vi "Untitled 2.vi"() -> ()   [LabVIEW 2016]
uses:
  <vilib>/AppBuilder/AB_API/PPL/NI_AB_API_PPL.lvclass
  <vilib>/AppBuilder/AB_API/Build/NI_AB_API_Build.lvclass
  <vilib>/AppBuilder/AB_API/SDIST/NI_AB_API_SDIST.lvclass
  C:/Program Files (x86)/National Instruments/LabVIEW 2016/vi.lib/AppBuilder/AB_API/Targetfile/NI_AB_API_Targetfile.lvclass
  C:/Program Files (x86)/National Instruments/LabVIEW 2016/vi.lib/AppBuilder/AB_API/Build/NI_AB_API_Build.lvclass
panel:
  in  "Destination":string
  out "Primary destination path":path
  out "error out":errorcluster
  out "Cluster":cluster{string, "Build":string, string}
  in  "Cancel":bool
  in  "OK":bool
  in  "Build":string(combo)
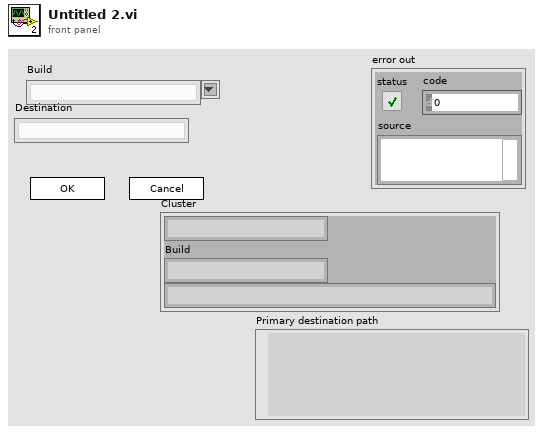
[diagram p1: front panel]
types:
  T1 = enum8{"Enabled", "Disabled", "Disabled and Grayed Out"}
  T2 = cluster{string, "Build":string, "Destination":string}
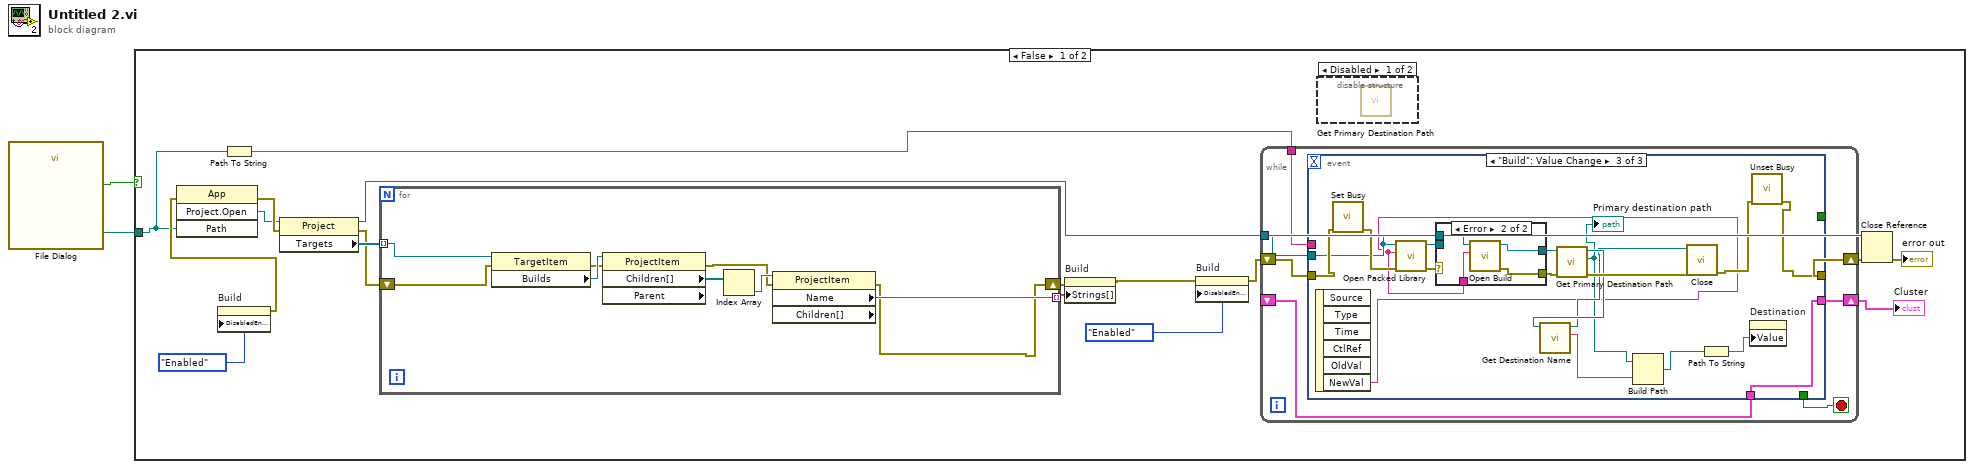
[diagram p0: block diagram]
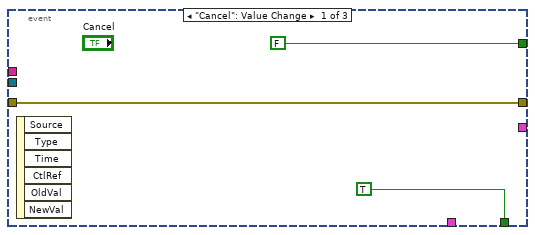
[diagram p2: hidden frame]
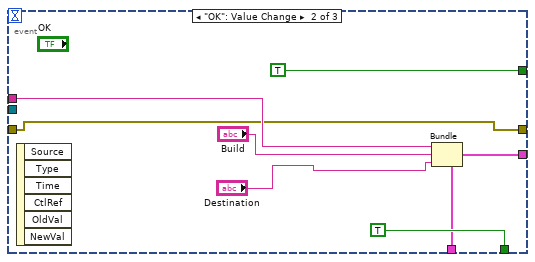
[diagram p3: hidden frame]
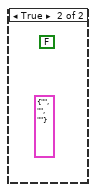
[diagram p6: hidden frame]
diagram:
  n1 = call "File Dialog"() -> ("selected path"=w1:path, "cancelled"=w2:bool)  [unwired: 12 in, 2 out]
  n2 = case shown="False" w2 {
    tunnel: w1 -> [w10 _]
    frame False {
      n3 = property on="Build" class="CmbBox"("DisabledEnum"=T1."Enabled" ("Disabled")) -> (error out=w15:errorcluster)  [unwired: 2 in, 1 out]
      n4 = invoke class="App" method="Project.Open"(error in=w15, "Path"=w10) -> (error out=w14:errorcluster, "Project:Open"=w7:refnum<vi>)  [unwired: 2 in, 2 out]
      n5 = Path To String(path=w10) -> (string=w9:string)
      n6 = property class="Project"(reference=w7, error in=w14) -> (reference out=w4:refnum<vi>, error out=w13:errorcluster, "Targets"=w19:refnum<vi>[])
      n7 = for {
        tunnel: w19 -> [w70] mode=indexing
        tunnel: [w66] -> w18 mode=indexing
        shift-right: [w62] -> w12
        shift-left: w13 -> [w65]
        n8 = property class="TargetItem"(reference=w70, error in=w65) -> (error out=w64:errorcluster, "Builds"=w69:refnum<vi>)  [unwired: 1 out]
        n9 = property class="ProjectItem" props=["Children[]", "Parent"](reference=w69, error in=w64) -> (error out=w63:errorcluster, "Children[]"=w68:refnum<vi>[])  [unwired: 2 out]
        n10 = Index Array(array=w68) -> (element=w67:refnum<vi>)  [unwired: 1 in]
        n11 = property class="ProjectItem" props=["Name", "Children[]"](reference=w67, error in=w63) -> (error out=w62:errorcluster, "Name"=w66:string)  [unwired: 2 out]
      }
      n12 = property on="Build" class="CmbBox"(error in=w12, "Strings[]"=w18) -> (error out=w5:errorcluster)  [unwired: 1 in, 1 out]
      n13 = property on="Build" class="CmbBox"(error in=w5, "DisabledEnum"=T1."Enabled" ("Disabled")) -> (error out=w11:errorcluster)  [unwired: 1 in, 1 out]
      n14 = while {
        tunnel: w9 -> [w25]
        tunnel: w4 -> [w22]
        shift-right: [w23] -> w6
        shift-left: w11 -> [w26]
        shift-right: [w24] -> w8
        shift-left: _ -> [w20]
        stop <- w21 stop-if-true
        n15 = event shown="[2] \"Build\": Value Change" {
          selector: _ -> [_ _ _]
          dyn-events: _ -> [_ _ _]
          timeout: _ -> [_ _ _]
          tunnel: w26 -> [w29 w34 w55]
          tunnel: [w29 w34 w53] -> w23
          tunnel: [FALSE ("Cancel") TRUE ("Cancel") _] -> _
          tunnel: w25 -> [_ w37 _]
          tunnel: [_ w35 w44] -> w24
          tunnel: w22 -> [_ _ w39]
          tunnel: [TRUE TRUE _] -> w21
          tunnel: w20 -> [_ w30 w44]
          event "Cancel": Value Change {
            n16 = event-data() -> ()  [unwired: 1 in, 6 out]
          }
          event "OK": Value Change {
            n17 = event-data() -> ()  [unwired: 1 in, 6 out]
            n18 = Bundle(cluster=w30, w37, "Build"="Build", "Destination"="Destination") -> (w35:T2)
          }
          event "Build": Value Change {
            n19 = event-data() -> ("NewVal"=w38:string)  [unwired: 1 in, 5 out]
            n20 = call <vilib>:"Set Busy.vi"("error in (no error)"=w55) -> ("error out"=w54:errorcluster)  [unwired: 9 in, 1 out]
            n21 = call <vilib>:"Open Packed Library.vi"("error in (no error)"=w54, "Build specification name"=w38, "Project Refnum"=w39) -> ("error out"=w43:errorcluster, "PPL out"=w40:refnum<class "NI_AB_API_PPL.lvclass">)  [unwired: 7 in]
            n22 = case shown="Error" w43 {
              selector: w43 -> [w57 _]
              tunnel: [w57 w61] -> w42
              tunnel: [w56 w60] -> w41
              tunnel: w40 -> [w56 _]
              tunnel: w39 -> [_ w59]
              tunnel: w38 -> [_ w58]
              frame No Error {
              }
              frame Error {
                n23 = call <vilib>:"Open Build.vi"("Build specification name"=w58, "Project Refnum"=w59) -> ("error out"=w61:errorcluster, "SDIST out"=w60:refnum<class "NI_AB_API_SDIST.lvclass">)  [unwired: 8 in]
              }
            }
            n24 = call-dynamic "Get Primary Destination Path.vi"("error in (no error)"=w42, "NI_AB_API_Build in"=w41) -> ("error out"=w51:errorcluster, "Primary destination path"=w47:path, "NI_AB_API_Build out"=w49:refnum<class "NI_AB_API_Build.lvclass">)  [unwired: 7 in]
            "Primary destination path" <- w47
            n25 = call-dynamic "Get Destination Name.vi"("NI_AB_API_Build in"=w49) -> ("Destination Name"=w45:string, "NI_AB_API_Build out"=w48:refnum<class "NI_AB_API_Build.lvclass">)  [unwired: 8 in, 1 out]
            n26 = Build Path(base path=w47, name or relative path=w45) -> (appended path=w46:path)
            n27 = call-dynamic "Close.vi"("error in (no error)"=w51, "NI_AB_API_Build in"=w48) -> ("error out"=w52:errorcluster)  [unwired: 9 in]
            n28 = Path To String(path=w46) -> (string=w50:string)
            n29 = property on="Destination" class="Str"("Value"=w50) -> ()  [unwired: 2 in, 2 out]
            n30 = call <vilib>:"Unset Busy.vi"("error in (no error)"=w52) -> ("error out"=w53:errorcluster)  [unwired: 10 in]
          }
        }
      }
      "Cluster" <- w8
      n31 = disable-structure shown="Disabled" {
        frame Disabled {
          n32 = call-dynamic "Get Primary Destination Path.vi"() -> ()  [unwired: 9 in, 3 out]
        }
        frame Enabled {
        }
      }
      n33 = Close Reference(reference=w4, error in (no error)=w6) -> (error out=→"error out":errorcluster)
    }
    frame True {
      (unwired) cluster{string, "Build":string, string} {"", "Build"="", ""}
      (unwired) FALSE ("Cancel")
    }
  }
